vi "Find Class in ProjectItem.vi"(8 "error in (no error)":errorcluster, 10 "Class Name":string="MyClass.lvclass", 11 "ProjectItem in":refnum<vi>) -> (0 "error out":errorcluster, 1 "Found?":bool, 2 "LVClass out":refnum<vi>, 3 "ProjectItem out":refnum<vi>)   [LabVIEW 2020, in "gRPC Scripting Tools.lvlib"]
uses:
  gRPC Scripting Tools.lvlib
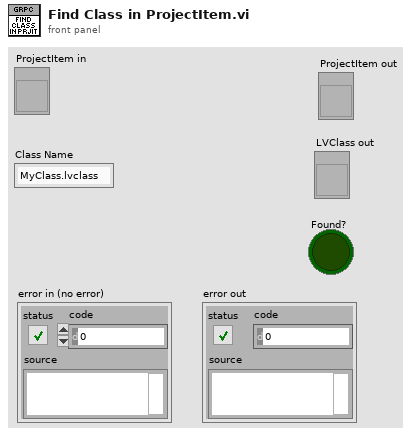
[diagram p1: front panel]
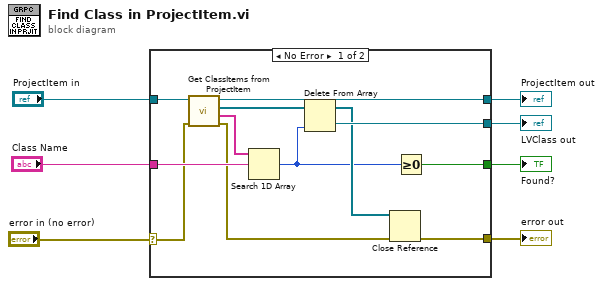
[diagram p0: block diagram]
diagram:
  n1 = case shown="No Error" "error in (no error)" {
    selector: "error in (no error)" -> [w16 w20]
    tunnel: [w10 w20] -> w7
    tunnel: "Class Name" -> [w19 _]
    tunnel: "ProjectItem in" -> [w17 w21]
    tunnel: [w15 w21] -> w3
    tunnel: [w14 _] -> w2
    tunnel: [w12 _] -> w1
    frame No Error {
      n2 = call "Get ClassItems from ProjectItem.vi"("error in (no error)"=w16, "ProjectItem in"=w17) -> ("error out"=w11:errorcluster, "Class Item Names"=w18:string[], "Class Items"=w13:refnum<vi>[], "ProjectItem out"=w15:refnum<vi>)  [unwired: 6 in]
      n3 = Search 1D Array(1D array=w18, element=w19) -> (index of element=w8:i32)  [unwired: 1 in]
      n4 = Delete From Array(array=w13, index=w8) -> (deleted portion=w12:refnum<vi>, array with subset deleted=w9:refnum<vi>[])  [unwired: 1 in]
      n5 = Close Reference(reference=w9, error in (no error)=w11) -> (error out=w10:errorcluster)
      n6 = Greater Or Equal To 0?(x=w8) -> (x >= 0?=w14:bool)
    }
    frame Error {
    }
  }
  "LVClass out" <- w1
  "error out" <- w7
  "ProjectItem out" <- w3
  "Found?" <- w2
